vi "SM Wait for Transition.vi"(7 "Timeout [ms]":i32=-1, 8 "error in (no error)":errorcluster, 11 "Event Registration Refnum":refnum<event-registration>) -> (0 "error out":errorcluster, 2 "Data":variant, 3 "Transition":T1)   [LabVIEW 2022 SP3, in "StateMachine.lvlib" / "HSE-State-Machine.lvlib"]
doc: "Waits for a Transition to occur in the duration of Timeout.\n____\nHAMPEL SOFTWARE ENGINEERING v2.6.0 (2023-12-19 10:54)"
uses:
  HSE-State-Machine.lvlib
  SM_Transitions.ctl
  SM Events/SM Request Transition Argument--cluster.ctl
  <vilib>/Hampel Software Engineering/HSE Logger/hse-logger.lvlib
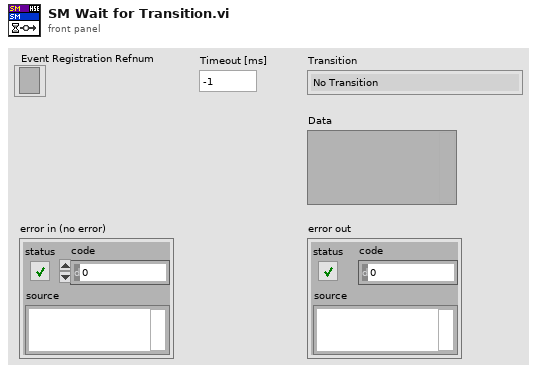
[diagram p1: front panel]
types:
  T1 = typedef "StateMachine.lvlib/HSE-State-Machine.lvlib/SM_Transitions.ctl" = enum16{"No Transition", "Exception", "Reset", "Initialization finished", "Process started", "Trigger detected", "Exit"}
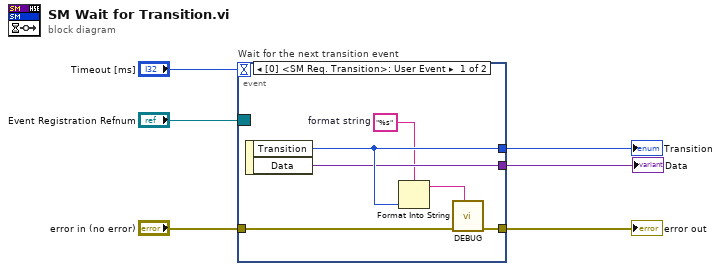
[diagram p0: block diagram]
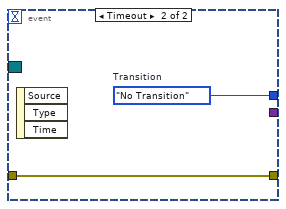
[diagram p2: hidden frame]
diagram:
  n1 = event "Wait for the next transition event" shown="[0] <SM Req. Transition>: User Event" {
    selector: "Event Registration Refnum" -> [_ _]
    dyn-events: _ -> [_ _]
    timeout: "Timeout [ms]" -> [_ _]
    tunnel: "error in (no error)" -> [w8 w13]
    tunnel: [w12 w14] -> w3
    tunnel: [w11 _] -> w5
    tunnel: [w7 w13] -> w2
    event User Event {
      w10 = "%s"  # format string
      n2 = event-data() -> ("Transition"=w12:T1, "Data"=w11:variant)  [unwired: 1 in]
      n3 = Format Into String(format string=w10, w12) -> (resulting string=w9:string)  [unwired: 2 in, 1 out]
      n4 = call <vilib>:"DEBUG.vi"("Message"=w9, "error in"=w8) -> ("error out"=w7:errorcluster)  [unwired: 9 in]
    }
    event Timeout {
      w14 = SM_Transitions."No Transition"  # Transition
      n5 = event-data() -> ()  [unwired: 1 in, 3 out]
    }
  }
  "Transition" <- w3
  "error out" <- w2
  "Data" <- w5
